vi "Controls - Controls.vi"(7 "Msg Chain":string, 8 "error in (no error)":errorcluster {"code" format="Error %.0f"}, 10 "Controls Docs":refnum<class "GUI Documentation.lvclass">[](array[class]), 11 "VIDoc Printer - Confluence In":refnum<class "VIDoc Printer - Confluence.lvclass">) -> (0 "error out":errorcluster {"code" format="Error %.0f"}, 3 "VIDoc Printer - Confluence Out":refnum<class "VIDoc Printer - Confluence.lvclass">)   [LabVIEW 2023, in "VIDoc Printer - Confluence.lvlib" / "VIDoc Printer - Confluence.lvclass"]
uses:
  VIDoc Printer - Confluence.lvclass
  C:/projects/DMC/Tooling/Git-Action-Service/Source/Documentation Generation/Printers/Printer/VIDoc Printer.lvclass
  Parsing/GUI Documentation/GUI Documentation.lvclass
  Confluence Formatting/Types/Format Combo Box.ctl
  Printer/VIDoc Printer.lvclass/VIDoc Printer.ctl
  Parsing/GUI Documentation/GUI Documentation.lvclass/GUI Documentation.ctl
  VIDoc Printer - Confluence.lvclass/VIDoc Printer - Confluence.ctl
  Parsing/GUI Documentation/Get VI Info.vi
  Parsing/GUI Documentation/Get Name.vi
  Printer/Accessors/Get Controls Settings - Controls Detail Level.vi
  Accessors/Get Ctrls Controls Expand.vi
  Printer/VIDoc Printer.lvclass
  UI Interaction/UI Interaction.lvclass
  Confluence Formatting/Confluence Formatting.lvlib
  C:/projects/DMC/Tooling/Git-Action-Service/Source/Documentation Generation/Printers/Confluence Printer/VIDoc Printer - Confluence.lvclass
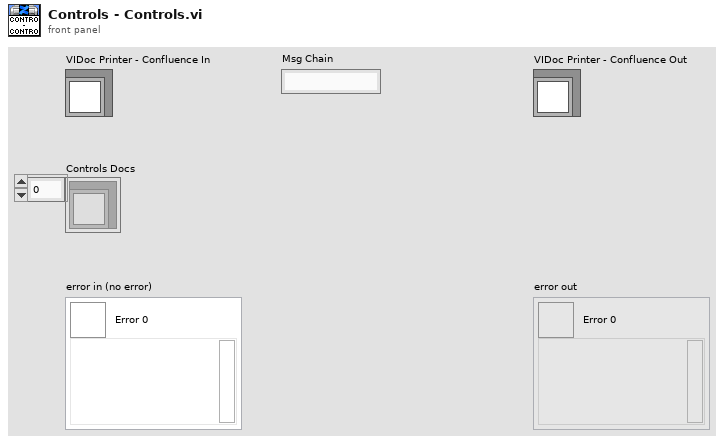
[diagram p1: front panel]
types:
  T1 = typedef "Confluence Formatting.lvlib/Format Combo Box.ctl" = string
  T2 = typedef "VIDoc Printer.lvlib/Printer Settings.lvclass/Detail Level Enum.ctl" = enum16{"None", "Minimal", "Standard", "Full"}
  T3 = typedef "VIDoc Parsing.lvlib/Method Spec Cluster.ctl" = cluster{"VI Type Ext":T4, "Name":string, "Path":path, "Get Conpane Image":T5, "Description":string, "Get Library Access Scope":enum32{"invalid scope", "public", "private", "protected", "community"}, "Dispatch":T6, "ContainsCompiledCode":bool, "Exec.IsReentrant":bool, "Exec.ReentrancyType":enum16{"Share clones between instances", "Preallocate clone for each instance"}, "ExecInlining":bool, "ExecInlineIfPossible":bool, "Auto Err Handling":bool, "CodeComplexity":sgl, "Bookmark Tags":string[], "Control VI Type":enum32{"not a control VI", "control", "typedef", "strict typedef"}, "Controls":T7[], "VI Type":enum32{"invalid VI type", "Standard VI", "Control VI", "Global VI", "Polymorphic VI", "Configuration VI", "SubSystem", "Facade VI", "Method VI", "Statechart Diagram VI"}, "Minimum Size":T9, "Front Panel Window:Title":string, "Front Panel Window:Behavior":enum32{"Invalid", "Default", "Floating", "Floating/Auto-Hide", "Modal"}, "Front Panel Window:Closeable":bool, "Must Override":bool, "Must Use Parent Implementation":bool, "VI Icon":T5, "Front Panel":T5, "History:Revision Number":u32, "Metrics:Total Data Size":u32, "Execution:Allow Debugging":bool, "Execution:Preferred Exec System":enum32{"invalid execution system", "user interface", "standard", "instrument i/o", "data acquisition", "other 1", "other 2", "same as caller"}, "Execution:Priority":enum32{"invalid priority", "background priority", "normal priority", "above normal priority", "high priority", "time critical priority", "subroutine"}, "BM Tag Text":string[], "Block Diagram":T5, "Structure Tree":T10[]}
  T4 = typedef "VIDoc Parsing.lvlib/VI Type Extended Enum.ctl" = enum16{"Unknown", "Class Method", "Class Accessor Get", "Class Accessor Set", "Class Control", "Library Method", "Library Control", "VI", "Control"}
  T5 = typedef "imagedata.ctl" = cluster{"image type":i32, "image depth":i32, "image":u8[], "mask":u8[], "colors":u32[], "Rectangle":cluster{"left":i16, "top":i16, "right":i16, "bottom":i16}}
  T6 = typedef "VIDoc Parsing.lvlib/Class Dispatch Type Enum.ctl" = enum16{"None", "Static", "Dynamic"}
  T7 = typedef "VIDoc Parsing.lvlib/Controls Info Cluster.ctl" = cluster{"Name":string, "Description":string, "Data Type":string, "Tip Strip":string, "UID":i32, "Image Data":T5, "ToggleKeyBind":T8, "Raw Label":string, "Raw Caption":string}
  T8 = typedef "LVKeyTypeDef.ctl" = cluster{"Focus":bool, "Control":bool, "Shift":bool, "Key":string}
  T9 = typedef "LVPointTypeDef.ctl" = cluster{"Horizontal":i16, "Vertical":i16}
  T10 = typedef "VIDoc Parsing.lvlib/Structure Reporter.lvlib/Tree Cluster.ctl" = cluster{"Object Class Name":string, "Labels":string[], "Child Tag":string, "Item Indent":i32, "Child Only?":bool, "Glyph Index":i32}
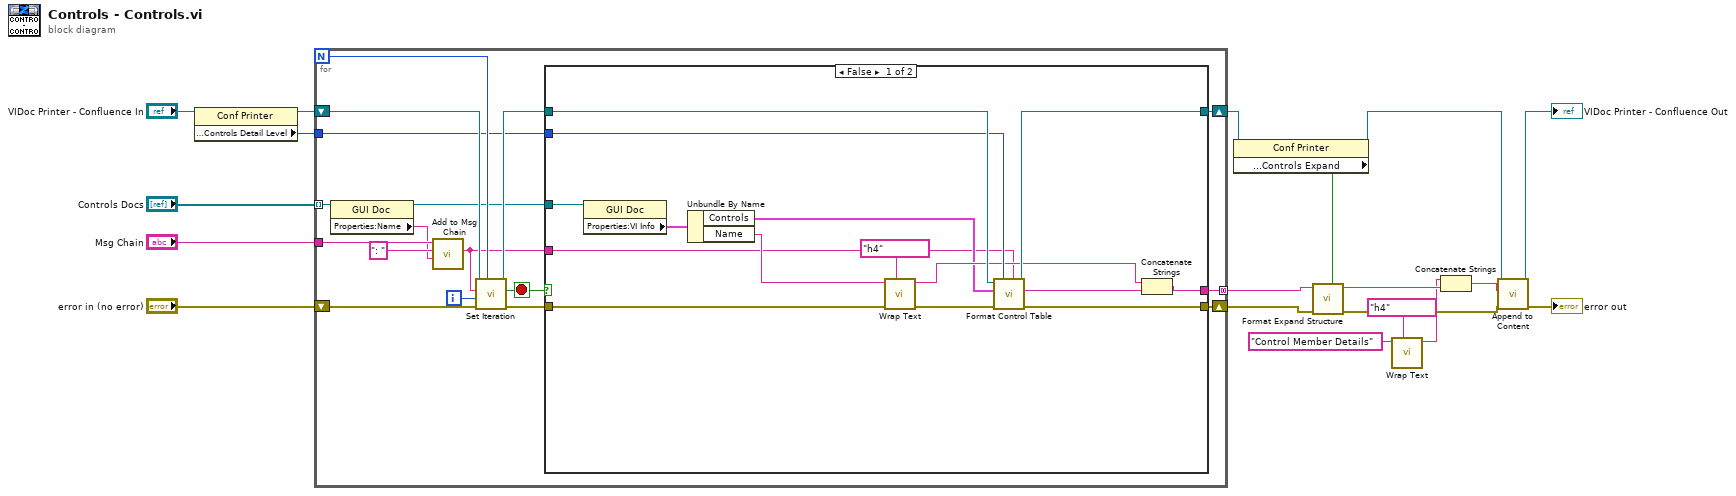
[diagram p0: block diagram]
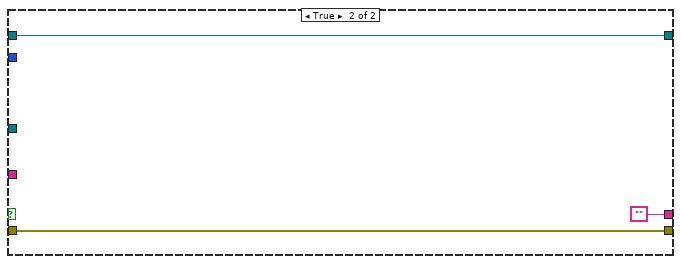
[diagram p2: hidden frame]
diagram:
  n1 = property class="Conf Printer"(reference="VIDoc Printer - Confluence In") -> (reference out=w19:refnum<class "VIDoc Printer - Confluence.lvclass">, "Properties:Settings:Control Members:Controls Detail Level"=w12:T2)  [unwired: 1 in, 1 out]
  n2 = for {
    N -> [w29]
    shift-right: [w35] -> w11
    shift-left: "error in (no error)" -> [w31]
    shift-right: [w36] -> w7
    shift-left: w19 -> [w33]
    tunnel: "Controls Docs" -> [w34] mode=indexing
    tunnel: "Msg Chain" -> [w26]
    tunnel: [w22] -> w9 mode=concatenating
    tunnel: w12 -> [w21]
    i -> [w28]
    stop <- w23 stop-if-true
    n3 = property class="GUI Doc"(reference=w34) -> (reference out=w25:refnum<class "GUI Documentation.lvclass">, "Properties:Name"=w24:string)  [unwired: 1 in, 1 out]
    n4 = call "Add to Msg Chain.vi"("New"=w24, "Separator (-)"=": ", "Msg Chain in"=w26) -> ("Msg Chain out"=w20:string)  [unwired: 8 in]
    n5 = call "Set Iteration.vi"("Progress Max"=w29, "error in (no error)"=w31, "Progress Value"=w28, "Message (No Message Update)"=w20, "VIDoc Printer In"=w33) -> ("error out"=w30:errorcluster, "Abort?"=w23:bool, "VIDoc Printer Out"=w32:refnum<class "VIDoc Printer - Confluence.lvclass">)  [unwired: 4 in]
    n6 = case shown="False" w23 {
      tunnel: [w51 w54] -> w36
      tunnel: [w50 w53] -> w35
      tunnel: w32 -> [w49 w54]
      tunnel: w30 -> [w48 w53]
      tunnel: w25 -> [w47 _]
      tunnel: [w46 ""] -> w22
      tunnel: w21 -> [w45 _]
      tunnel: w20 -> [w37 _]
      frame False {
        n7 = property class="GUI Doc"(reference=w47) -> ("Properties:VI Info"=w42:T3)  [unwired: 1 in, 2 out]
        n8 = Unbundle By Name(w42) -> ("Controls"=w40:T7[], "Name"=w38:string)
        n9 = call "Wrap Text.vi"("Formatting"=T1 "h4", "Error in"=w48, "String"=w38) -> ("Error out"=w43:errorcluster, "Wrapped String"=w41:string)  [unwired: 7 in]
        n10 = call "Format Control Table.vi"("Msg Chain in"=w37, "Controls Opt"=w45, "error in (no error)"=w43, "Controls"=w40, "VIDoc Printer - Confluence In"=w49) -> ("error out"=w50:errorcluster, "Table"=w39:string, "VIDoc Printer - Confluence Out"=w51:refnum<class "VIDoc Printer - Confluence.lvclass">)  [unwired: 4 in]
        n11 = Concatenate Strings(w41, w39) -> (w46:string)
      }
      frame True {
      }
    }
  }
  n12 = property class="Conf Printer"(reference=w7) -> (reference out=w6:refnum<class "VIDoc Printer - Confluence.lvclass">, "Properties:Expand?:Control:Controls Expand"=w5:bool)  [unwired: 1 in, 1 out]
  n13 = call "Format Expand Structure.vi"("Enable? (T)"=w5, "Error in"=w11, "Content"=w9) -> ("Error out"=w10:errorcluster, "Expand String"=w8:string)  [unwired: 7 in]
  n14 = call "Wrap Text.vi"("Formatting"=T1 "h4", "String"="Control Member Details") -> ("Wrapped String"=w1:string)  [unwired: 8 in, 1 out]
  n15 = Concatenate Strings(w1, w8) -> (w2:string)
  n16 = call "Append to Content.vi"("error in (no error)"=w10, "Content"=w2, "VIDoc Printer - Confluence In"=w6) -> ("error out"=→"error out":errorcluster, "VIDoc Printer - Confluence Out"=→"VIDoc Printer - Confluence Out":refnum<class "VIDoc Printer - Confluence.lvclass">)  [unwired: 7 in]
